vi "Log Data.vi"(7 "Command":enum16{"Initilalize", "Write", "Close"}(ring)=enum."Close", 8 "error in (no error)":errorcluster, 9 "Array":string[](array[string]), 10 "Boolean":bool, 11 "file path":path) -> (0 "error out":errorcluster)   [LabVIEW 2013]
doc: "This subVI writes the data to the Boiler Log.txt file.\nItem that has to be logged in the file are-\n-Time String: Absolute date and time at event\n-Event String: A string value which is different for different state\n-Event data String: It could be \n1.Zero\n2.Elapsed time\n3.True\n4.False."
uses:
  <vilib>/Utility/file.llb/Write To Spreadsheet File (string).vi
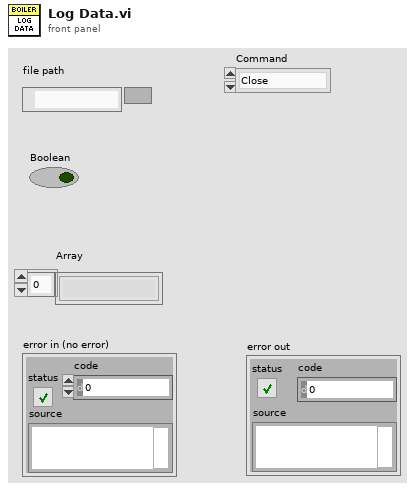
[diagram p1: front panel]
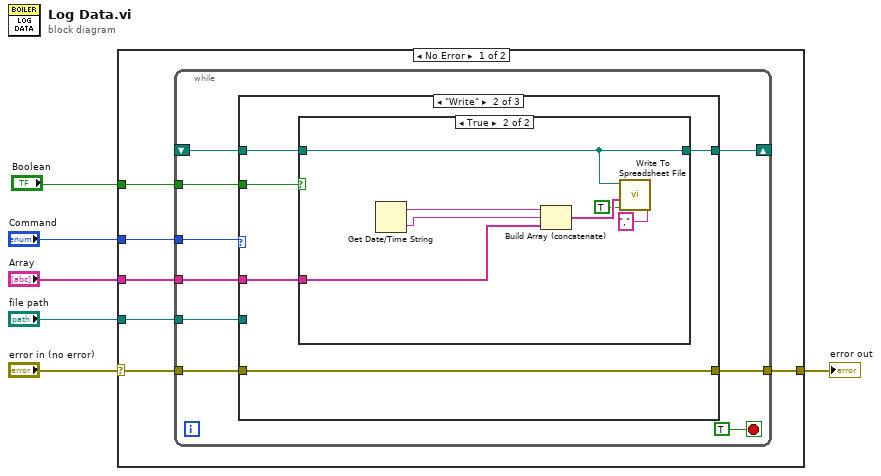
[diagram p0: block diagram]
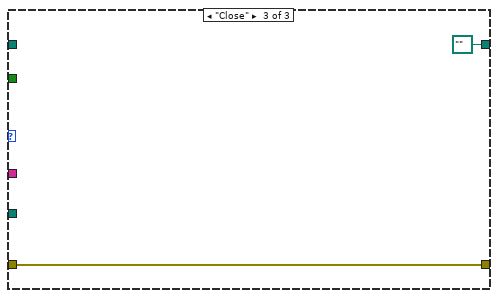
[diagram p4: hidden frame]
diagram:
  n1 = case shown="No Error" "error in (no error)" {
    selector: "error in (no error)" -> [w9 w39]
    tunnel: "Array" -> [w12 _]
    tunnel: "file path" -> [w11 _]
    tunnel: [w10 w39] -> w6
    tunnel: "Command" -> [w8 _]
    tunnel: "Boolean" -> [w7 _]
    frame No Error {
      n2 = while {
        tunnel: w12 -> [w21]
        tunnel: w11 -> [w20]
        tunnel: [w19] -> w10
        tunnel: w9 -> [w18]
        tunnel: w8 -> [w17]
        shift-right: [w16] -> _
        shift-left: _ -> [w15]
        tunnel: w7 -> [w13]
        stop <- TRUE stop-if-true
        n3 = case shown="\"Write\"" w17 {
          tunnel: w21 -> [_ w28 _]
          tunnel: w20 -> [w23 _ _]
          tunnel: w18 -> [w22 w27 w37]
          tunnel: [w22 w27 w37] -> w19
          tunnel: [w23 w24 path "" ("file path (dialog if empty)")] -> w16
          tunnel: w15 -> [_ w26 _]
          tunnel: w13 -> [_ w25 _]
          frame "Initilalize", Default {
          }
          frame "Write" {
            n4 = case shown="True" w25 {
              tunnel: w28 -> [_ w36]
              tunnel: w26 -> [w29 w30]
              tunnel: [w29 w30] -> w24
              frame False {
              }
              frame True {
                n5 = Get Date/Time String() -> (date string=w35:string, time string=w34:string)  [unwired: 3 in]
                n6 = Build Array (concatenate)(w35, w34, w36) -> (w33:string[])
                n7 = call-poly <vilib>:"Write To Spreadsheet File.vi"("delimiter (\\t)"="," ("delimiter (\\t)"), "append to file? (new file:F)"=TRUE, "1D data"=w33, "file path (dialog if empty)"=w30) -> ()  [unwired: 4 in, 1 out]
              }
            }
          }
          frame "Close" {
          }
        }
      }
    }
    frame Error {
    }
  }
  "error out" <- w6
